vi "Send.vi"(8 "error in (no error)":errorcluster, 10 "data":string, 11 "refnum in":refnum<visa-resource-name>) -> (0 "error out":errorcluster, 3 "refnum out":refnum<visa-resource-name>)   [LabVIEW 2020, in "Korad KA3305P.lvlib"]
uses:
  Korad KA3305P.lvlib
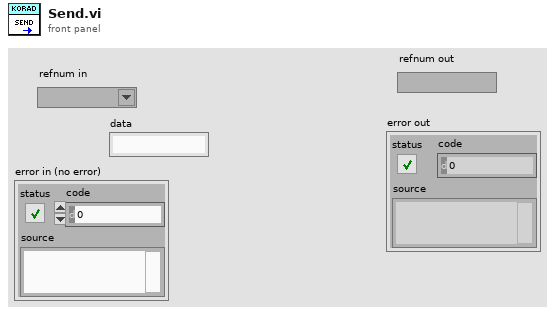
[diagram p1: front panel]
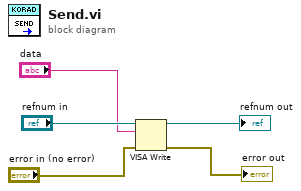
[diagram p0: block diagram]
diagram:
  n1 = VISA Write(VISA resource name="refnum in", write buffer="data", error in (no error)="error in (no error)") -> (VISA resource name out=→"refnum out":refnum<visa-resource-name>, error out=→"error out":errorcluster)  [unwired: 1 out]
